vi "Init.vi"() -> (0 "error out":errorcluster, 3 "Queue Msg Type Strategy out":refnum<class "Queue Msg Type Strategy.lvclass">)   [LabVIEW 2021, in "jettl.lvlib" / "Msg Type Strategy.lvlib" / "Queue Msg Type Strategy.lvclass"]
uses:
  Queue Msg Type Strategy.lvclass
  Msg Strategy/Msg Strategy.lvclass
  Queue Msg Type Strategy.lvclass/Queue Msg Type Strategy.ctl
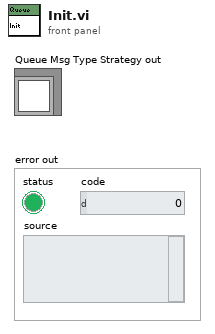
[diagram p1: front panel]
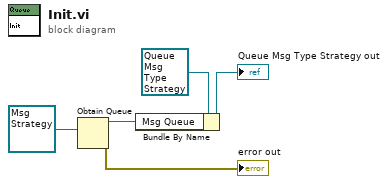
[diagram p0: block diagram]
diagram:
  n1 = Obtain Queue(element data type=refnum<class "Msg Strategy.lvclass"> refnum ("Msg.lvclass")) -> (queue out=w1:refnum<queue>, error out=→"error out":errorcluster)  [unwired: 4 in, 1 out]
  n2 = Bundle By Name(cluster=refnum<class "Queue Msg Type Strategy.lvclass"> refnum ("Queue Msg Type Strategy out"), "Msg Queue"=w1) -> (→"Queue Msg Type Strategy out":refnum<class "Queue Msg Type Strategy.lvclass">)
